vi "FTW-Dataflow-Parallelize.vi"(1 "Parallelize?":bool=TRUE) -> (0 "Parallel Instances":i32)   [LabVIEW 2014]
panel:
  # "Inputs"
  # "Outputs"
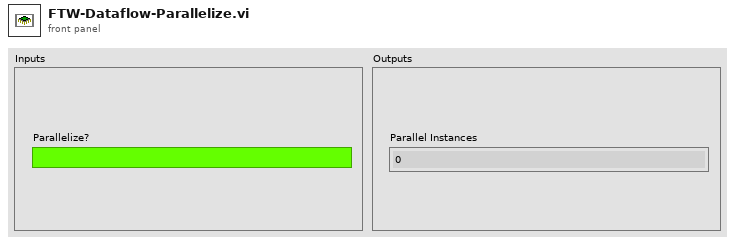
[diagram p1: front panel]
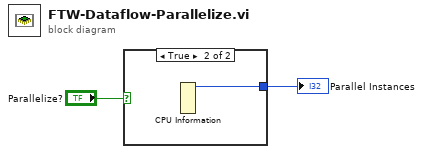
[diagram p0: block diagram]
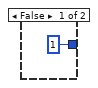
[diagram p2: hidden frame]
diagram:
  n1 = case shown="True" "Parallelize?" {
    tunnel: [1 ("# of logical processors") w4] -> w1
    frame False {
    }
    frame True {
      n2 = CPU Information() -> (4:w4:i32)  [unwired: 3 out]
    }
  }
  "Parallel Instances" <- w1
